vi "draw_track7_image.vi"(2 "GOALpos":cluster{"X":sgl, "Y":sgl}[](array[cluster]), 3 "角度阈值":dbl=60.0 format="%#_13g", 4 "距离阈值":dbl=1000.0 format="%#_13g", 5 "bin_billard":T1, 6 "color_billard":T1) -> (0 "color_billard 2":T1, 1 "大小":i32)   [LabVIEW 2018]
uses:
  <vilib>/vision/Shape Detection.llb/ShapeDetectionMatchOptions.ctl
  <vilib>/vision/Pattern Matching.llb/IMAQ Match Range Setting.ctl
  <vilib>/vision/Image Controls.llb/IMAQ Image.ctl
  <vilib>/vision/NI_Vision_Development_Module.lvlib
panel:
  in  "Match Options":T2={"Rotation"=TRUE, "Scale"=FALSE, "Occlusion"=FALSE, "Range Settings"=[]} {"Range Settings"."Match Constraints" items=["Rotation Angle (degrees)", "Scale Factor (%)", "Occlusion (%)"]}
  out "endX":dbl format="%#_13g"
  out "endY":dbl format="%#_13g"
  # "Range"
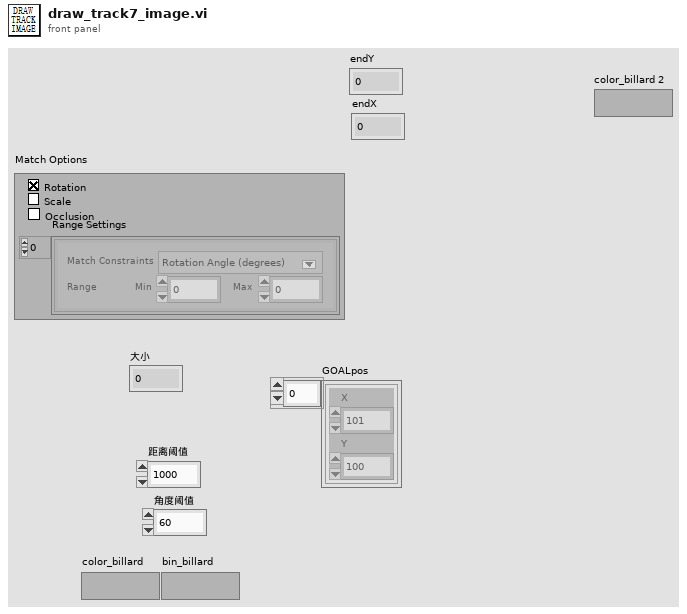
[diagram p1: front panel]
types:
  T1 = typedef "IMAQ Image.ctl" = refnum<image>
  T2 = typedef "ShapeDetectionMatchOptions.ctl" = cluster{"Rotation":bool, "Scale":bool, "Occlusion":bool, "Range Settings":T3[]}
  T3 = typedef "IMAQ Match Range Setting.ctl" = cluster{"Match Constraints":u32, "Min":dbl, "Max":dbl}
  T4 = cluster{"Position":cluster{"X":sgl, "Y":sgl}, "Radius":dbl, "Score":dbl}[]
  T5 = cluster{"Position":cluster{"X":sgl, "Y":sgl}, "Radius":dbl, "Score":dbl}
  T6 = cluster{i32, i32, "X Resolution":i32, "Y Resolution":i32}
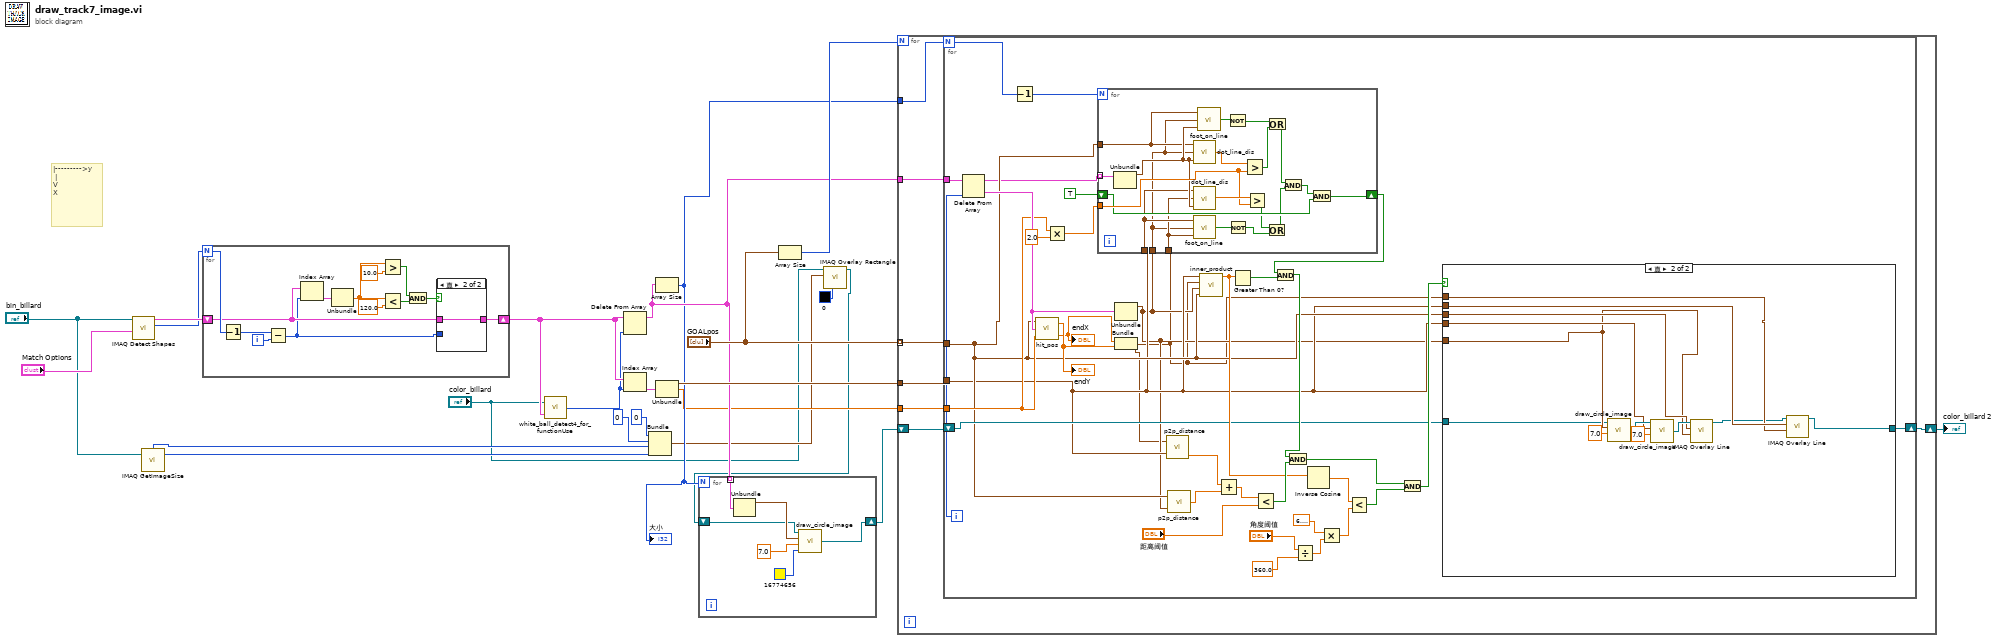
[diagram p0: block diagram]
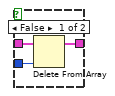
[diagram p3: hidden frame]
diagram:
  # "|--------->y\n |\nV\nX"
  n1 = call-poly "IMAQ Detect Shapes"("Match Options"="Match Options", "Image"="bin_billard") -> ("Number of Matches Returned"=w21:i32, "Circles"=w22:T4)  [unwired: 7 in, 1 out]
  n2 = call "IMAQ GetImageSize"("Image"="bin_billard") -> ("Y Resolution"=w11:i32, "X Resolution"=w10:i32)  [unwired: 3 in, 1 out]
  n3 = for {
    N: w21 -> [w31]
    shift-right: [w25] -> w16
    shift-left: w22 -> [w26]
    i -> [w29]
    n4 = Decrement(x=w31) -> (x-1=w30:i32)
    n5 = Subtract(x=w30, y=w29) -> (x-y=w24:i32)
    n6 = Index Array(array=w26, index=w24) -> (element=w28:T5)
    n7 = Unbundle(w28) -> ("Radius"=w35:dbl)  [unwired: 2 out]
    n8 = Greater?(x=w35, y=10.0) -> (0:w33:bool)
    n9 = Less?(x=w35, y=120.0) -> (x < y?=w32:bool)
    n10 = And(x=w33, y=w32) -> (x .and. y?=w27:bool)
    n11 = case shown="真" w27 {
      tunnel: w26 -> [w39 w40]
      tunnel: [w38 w40] -> w25
      tunnel: w24 -> [w37 _]
      frame False {
        n12 = Delete From Array(array=w39, index=w37) -> (array with subset deleted=w38:T4)  [unwired: 1 in, 1 out]
      }
      frame True {
      }
    }
  }
  n13 = call "white_ball_detect4_for_functionUse.vi"("Circles"=w16, "color_billard"="color_billard") -> ("白球所在(已处理的)数组位置"=w15:i32)
  n14 = Delete From Array(array=w16, index=w15) -> (array with subset deleted=w9:T4)  [unwired: 1 in, 1 out]
  n15 = Index Array(array=w16, index=w15) -> (element=w20:T5)
  n16 = Bundle(0, 0, "X Resolution"=w10, "Y Resolution"=w11) -> (w5:T6)  [unwired: 1 in]
  n17 = Array Size(array=w9) -> (size(s)=w8:i32)
  "大小" <- w8
  n18 = Unbundle(w20) -> ("Position"=w19:cluster{"X":sgl, "Y":sgl}, "Radius"=w7:dbl)  [unwired: 1 out]
  n19 = Array Size(array="GOALpos") -> (size(s)=w17:i32)
  n20 = call "IMAQ Overlay Rectangle"("Color"=u32 0, "Rectangle"=w5, "Image"="color_billard") -> ("Image Out"=w2:T1)  [unwired: 7 in, 1 out]
  n21 = for {
    N: w8 -> [_]
    tunnel: w9 -> [w46] mode=indexing
    shift-right: [w43] -> w1
    shift-left: w2 -> [w44]
    n22 = Unbundle(w46) -> ("Position"=w45:cluster{"X":sgl, "Y":sgl})  [unwired: 2 out]
    n23 = call "draw_circle_image.vi"("Color"=u32 16774656, "radius"=7.0, "Position"=w45, "Image"=w44) -> ("Image Out"=w43:T1)
  }
  n24 = for {
    N: w17 -> [_]
    tunnel: w19 -> [w53]
    tunnel: w8 -> [w52]
    tunnel: "GOALpos" -> [w51] mode=indexing
    tunnel: w9 -> [w50]
    tunnel: w7 -> [w49]
    shift-right: [w48] -> w6
    shift-left: w1 -> [w47]
    n25 = for {
      N: w52 -> [w87]
      tunnel: w53 -> [w57]
      tunnel: w51 -> [w61]
      tunnel: w50 -> [w84]
      tunnel: w49 -> [w64]
      shift-right: [w66] -> w48
      shift-left: w47 -> [w65]
      i -> [w85]
      n26 = Delete From Array(array=w84, index=w85) -> (deleted portion=w83:T5, array with subset deleted=w60:T4)  [unwired: 1 in]
      n27 = Decrement(x=w87) -> (x-1=w62:i32)
      n28 = call "hit_pos.vi"("radius"=w64, "TARGET Circle Descriptor"=w83, "GOALpos"=w61) -> ("endX"=w88:dbl, "endY"=w89:dbl)
      "endY" <- w89
      "endX" <- w88
      n29 = Multiply(x=w64, y=2.0) -> (x*y=w58:dbl)
      n30 = Unbundle(w83) -> ("Position"=w56:cluster{"X":sgl, "Y":sgl})  [unwired: 2 out]
      n31 = Bundle("endX"=w88, "endY"=w89) -> (w55:cluster{"endX":dbl, "endY":dbl})  [unwired: 1 in]
      n32 = for {
        N: w62 -> [_]
        tunnel: w61 -> [w101]
        tunnel: w60 -> [w109] mode=indexing
        tunnel: w56 -> [w92]
        tunnel: w57 -> [w99]
        tunnel: w55 -> [w98]
        tunnel: w58 -> [w106]
        shift-right: [w103] -> w54
        shift-left: TRUE -> [w104]
        n33 = Unbundle(w109) -> ("Position"=w102:cluster{"X":sgl, "Y":sgl})  [unwired: 2 out]
        n34 = call "dot_line_dis.vi"("dot pos"=w102, "line end"=w92, "line start"=w101) -> ("distance"=w108:sgl)
        n35 = call "dot_line_dis.vi"("dot pos"=w102, "line end"=w98, "line start"=w99) -> ("distance"=w107:sgl)
        n36 = call "foot_on_line.vi"("dot"=w98, "line end"=w92, "line start"=w99) -> ("foot on line？"=w96:bool)
        n37 = call "foot_on_line.vi"("dot"=w102, "line end"=w92, "line start"=w101) -> ("foot on line？"=w97:bool)
        n38 = Not(x=w97) -> (.not. x?=w91:bool)
        n39 = Not(x=w96) -> (.not. x?=w90:bool)
        n40 = Greater?(x=w108, y=w106) -> (0:w100:bool)
        n41 = Greater?(x=w107, y=w106) -> (0:w95:bool)
        n42 = Or(x=w95, y=w90) -> (x .or. y?=w93:bool)
        n43 = Or(x=w91, y=w100) -> (x .or. y?=w94:bool)
        n44 = And(x=w94, y=w93) -> (x .and. y?=w105:bool)
        n45 = And(x=w105, y=w104) -> (x .and. y?=w103:bool)
      }
      n46 = call "p2p_distance.vi"("point2"=w57, "point1"=w55) -> ("poit2poit_dis"=w82:dbl)
      n47 = call "p2p_distance.vi"("point2"=w56, "point1"=w61) -> ("poit2poit_dis"=w81:dbl)
      n48 = call "inner_product.vi"("L2ENDpos"=w61, "L2STARTpos"=w56, "L1ENDpos"=w55, "L1STARTpos"=w57) -> ("数值"=w76:dbl)  [unwired: 7 in]
      n49 = Add(x=w82, y=w81) -> (x+y=w80:dbl)
      n50 = Greater Than 0?(x=w76) -> (x > 0?=w86:bool)
      n51 = Less?(x=w80, y="距离阈值") -> (x < y?=w77:bool)
      n52 = And(x=w54, y=w86) -> (x .and. y?=w78:bool)
      n53 = And(x=w78, y=w77) -> (x .and. y?=w73:bool)
      n54 = Divide(x="角度阈值", y=360.0) -> (x/y=w69:dbl)
      n55 = Inverse Cosine(1:w76) -> (0:w75:dbl)
      n56 = Multiply(x=6.283185307179586, y=w69) -> (x*y=w70:dbl)
      n57 = Less?(x=w75, y=w70) -> (x < y?=w74:bool)
      n58 = And(x=w73, y=w74) -> (x .and. y?=w72:bool)
      n59 = case shown="真" w72 {
        tunnel: w61 -> [_ w119]
        tunnel: w56 -> [_ w118]
        tunnel: w57 -> [_ w117]
        tunnel: w55 -> [_ w116]
        tunnel: w57 -> [_ w121]
        tunnel: [w110 w114] -> w66
        tunnel: w65 -> [w110 w111]
        frame False {
        }
        frame True {
          n60 = call "draw_circle_image.vi"("radius"=7.0, "Position"=w118, "Image"=w111) -> ("Image Out"=w122:T1)  [unwired: 1 in]
          n61 = call "draw_circle_image.vi"("radius"=7.0, "Position"=w121, "Image"=w122) -> ("Image Out"=w120:T1)  [unwired: 1 in]
          n62 = call "IMAQ Overlay Line"("End Point"=w118, "Start Point"=w119, "Image"=w120) -> ("Image Out"=w115:T1)  [unwired: 7 in, 1 out]
          n63 = call "IMAQ Overlay Line"("End Point"=w116, "Start Point"=w117, "Image"=w115) -> ("Image Out"=w114:T1)  [unwired: 7 in, 1 out]
        }
      }
    }
  }
  "color_billard 2" <- w6
